vi "RT Inhibit Bus B - Single RT.vi"(8 "error in (no error)":errorcluster, 11 "1553 Unit Test in":refnum<class "Remote Terminal.lvclass">) -> (0 "error out":errorcluster, 3 "1553 Unit Test out":refnum<class "Remote Terminal.lvclass">)   [LabVIEW 2020, in "Unit Tests.lvlib" / "Remote Terminal.lvclass"]
uses:
  Remote Terminal.lvclass
  Remote Terminal/TypeDefs/RT Configuration.ctl
  Remote Terminal/TypeDefs/RT-RT Timeout.ctl
  Remote Terminal/TypeDefs/Mode Code 17 Sync Configuration.ctl
  Remote Terminal/TypeDefs/RT Timetag Configuration.ctl
  Remote Terminal/TypeDefs/RT Command Config.ctl
  Frames & Messages/TypeDefs/Command Type.ctl
  Frames & Messages/TypeDefs/Command SubAddress.ctl
  Frames & Messages/TypeDefs/Command Word Count.ctl
  Frames & Messages/TypeDefs/Simplified Parameter Data Table.ctl
  Frames & Messages/TypeDefs/Scaling Information.ctl
  Remote Terminal.lvclass/Remote Terminal.ctl
  Remote Terminal/Remote Terminal.lvclass
  C:/Users/MattJ/Desktop/git/bci-1553-labview-api/src/1553 SubComponent/1553 SubComponent.lvclass
  <vilib>/addons/_JKI Toolkits/Caraya/classes/Assert/Assert True.vi
  1553 Session/1553 Session.lvclass
  Dependencies/FPGA Interface/FPGA Interface.lvclass
  <vilib>/addons/_JKI Toolkits/Caraya/classes/Test/Test.lvclass
  BCI-1553 API.lvlib
  1553 Component/1553 Component.lvclass
  <vilib>/addons/_JKI Toolkits/Caraya/classes/Assert/Assert.lvclass
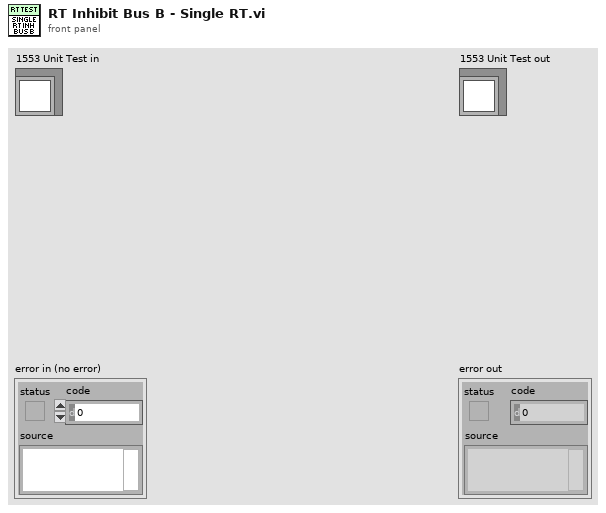
[diagram p1: front panel]
types:
  T1 = typedef "BCI-1553 API.lvlib/Remote Terminal.lvclass/RT Command Config.ctl" = cluster{"Command Type":T2, "SubAddress":T3, "Word Count\\Mode Code":T4, "Initial Data":u16[], "Data Fields":T5[]}
  T2 = typedef "BCI-1553 API.lvlib/Command Type.ctl" = enum16{"Transmit", "Receive"}
  T3 = typedef "BCI-1553 API.lvlib/Command SubAddress.ctl" = enum16{"Mode Code", "1", "2", "3", "4", "5", "6", "7", "8", "9", "10", "11", "12", "13", "14", "15", "16", "17", "18", "19", "20", "21", "22", "23", "24", "25", "26", "27", "28", "29", "30"}
  T4 = typedef "BCI-1553 API.lvlib/Command Word Count.ctl" = enum16{"1", "2", "3", "4", "5", "6", "7", "8", "9", "10", "11", "12", "13", "14", "15", "16", "17", "18", "19", "20", "21", "22", "23", "24", "25", "26", "27", "28", "29", "30", "31", "32"}
  T5 = typedef "BCI-1553 API.lvlib/Simplified Parameter Data Table.ctl" = cluster{"Parameter Name":string, "Base Word":u16, "Scaling Info":T6}
  T6 = typedef "BCI-1553 API.lvlib/Scaling Information.ctl" = cluster{"Bit Offset":i32, "Bit Count":i32, "LSB Resolution":dbl, "2's Complement":bool, "Big Endian":bool, "Sign Bit":bool}
  T7 = typedef "BCI-1553 API.lvlib/Remote Terminal.lvclass/RT Configuration.ctl" = cluster{"RT-RT Timeout":T8, "Inhibit Bus A":bool, "Inhibit Bus B":bool, "Broadcast CMD Invalid":bool, "UnDef MCs Invalid":bool, "Notice 2 Data Storage":bool, "SMCP":bool, "Temp RX Buffer":bool, "Alt BIT Enable":bool, "Auto Bus Shutdown":bool, "MC 16 SR Reset":bool, "MC 17 Sync":T9, "MC 8 Reset":bool, "Remote Terminal Timetag Config":T10}
  T8 = typedef "BCI-1553 API.lvlib/Remote Terminal.lvclass/RT-RT Timeout.ctl" = enum16{"57us", "62us", "100us", "180us"}
  T9 = typedef "BCI-1553 API.lvlib/Remote Terminal.lvclass/Mode Code 17 Sync Configuration.ctl" = enum16{"Sync if Bit 0 = 1", "Sync if Bit 0 = 0", "Sync Unconditionally"}
  T10 = typedef "BCI-1553 API.lvlib/Remote Terminal.lvclass/RT Timetag Configuration.ctl" = enum16{"Disabled", "2us", "4us", "8us", "16us", "32us", "64us"}
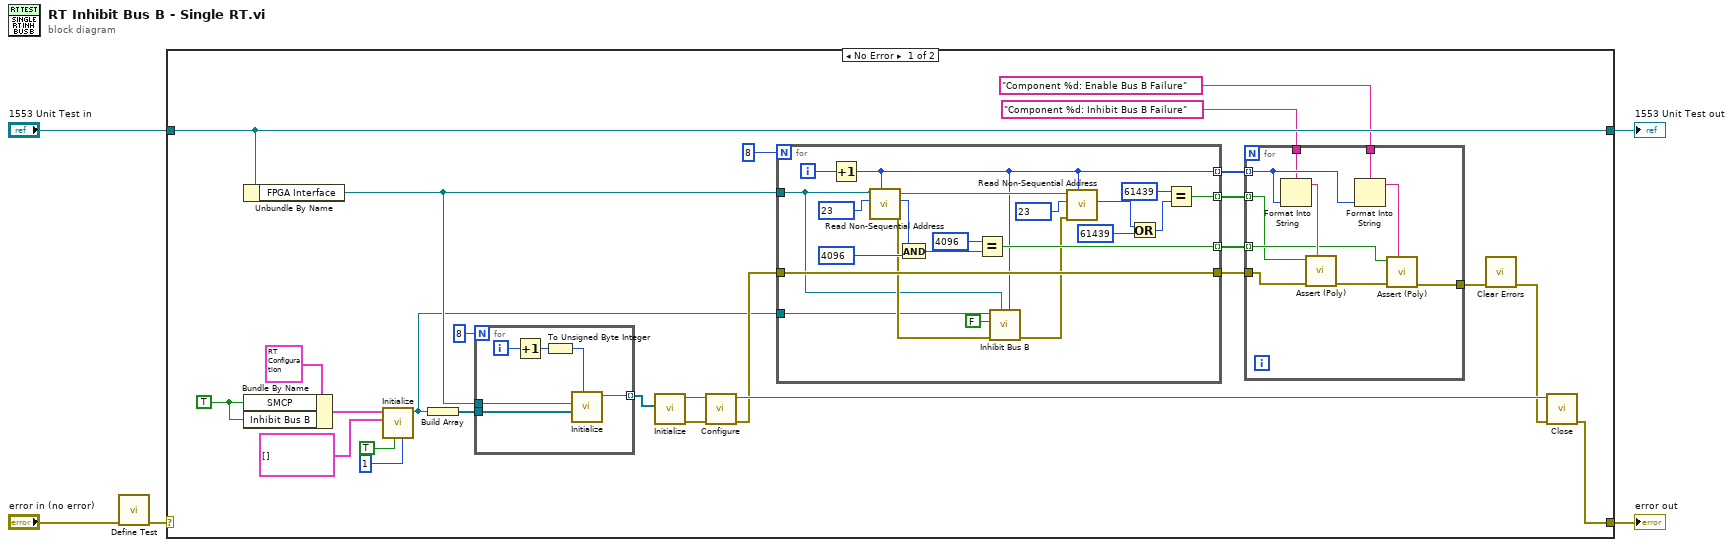
[diagram p0: block diagram]
diagram:
  n1 = call <vilib>:"Define Test.vi"("error in (no error)"="error in (no error)") -> ("error out"=w1:errorcluster)  [unwired: 9 in, 1 out]
  n2 = case shown="No Error" w1 {
    selector: w1 -> [_ w69]
    tunnel: [w14 w69] -> w5
    tunnel: [w25 w68] -> w3
    tunnel: "1553 Unit Test in" -> [w25 w68]
    frame No Error {
      w27 = TRUE ("SMCP")
      n3 = Unbundle By Name(w25) -> ("FPGA Interface"=w12:refnum<class "FPGA Interface.lvclass">)
      n4 = Bundle By Name(cluster=T7 {"RT-RT Timeout"=enum."57us", "Inhibit Bus A"=FALSE, "Inhibit Bus B"=FALSE, "Broadcast CMD Invalid"=FALSE, "UnDef MCs Invalid"=FALSE, "Notice 2 Data Storage"=FALSE, "SMCP"=FALSE, "Temp RX Buffer"=FALSE, "Alt BIT Enable"=FALSE, "Auto Bus Shutdown"=FALSE, "MC 16 SR Reset"=FALSE, "MC 17 Sync"=enum."Sync if Bit 0 = 1", "MC 8 Reset"=FALSE, "Remote Terminal Timetag Config"=enum."Disabled"} ("RT Configuration"), "SMCP"=w27, "Inhibit Bus B"=w27) -> (w30:T7)
      n5 = call "Initialize.vi"("Terminal Address"=u8 1 ("RT Address (0-30)"), "RT 1?"=TRUE, "RT Commands"=T1[] [], "RT Configuration"=w30) -> ("Remote Terminal out"=w10:refnum<class "Remote Terminal.lvclass">)  [unwired: 6 in, 1 out]
      n6 = Build Array(w10) -> (w23:refnum<class "Remote Terminal.lvclass">[])
      n7 = for {
        N: 8 -> [_]
        tunnel: [w65] -> w22 mode=indexing
        tunnel: w23 -> [w64]
        tunnel: w12 -> [w63]
        i -> [w67]
        n8 = Increment(x=w67) -> (x+1=w62:i32)
        n9 = To Unsigned Byte Integer(number=w62) -> (unsigned 8bit integer=w66:u8)
        n10 = call "Initialize.vi"("Component ID (1-8)"=w66, "SubComponents"=w64, "FPGA Interface"=w63) -> ("1553 Component out"=w65:refnum<class "1553 Component.lvclass">)  [unwired: 7 in, 1 out]
      }
      n11 = call "Initialize.vi"("Components"=w22) -> ("error out"=w20:errorcluster, "1553 Board out"=w21:refnum<class "1553 Session.lvclass">)  [unwired: 9 in]
      n12 = call-dynamic "Configure.vi"("error in (no error)"=w20, "1553 Board in"=w21) -> ("error out"=w11:errorcluster, "1553 Board out"=w17:refnum<class "1553 Session.lvclass">)  [unwired: 8 in]
      n13 = for {
        N: 8 -> [_]
        tunnel: w11 -> [w45]
        tunnel: [w45] -> w9
        tunnel: w12 -> [w40]
        tunnel: [w44] -> w8 mode=indexing
        tunnel: [w39] -> w6 mode=indexing
        tunnel: w10 -> [w42]
        tunnel: [w35] -> w7 mode=indexing
        i -> [w46]
        n14 = Increment(x=w46) -> (x+1=w39:i32)
        n15 = call-dynamic "Read Non-Sequential Address.vi"("Target IC (1-8)"=w39, "Address"=u16 23, "FPGA Interface in"=w40) -> ("error out"=w43:errorcluster, "Data"=w47:u16)  [unwired: 7 in]
        n16 = And(x=w47, y=u16 4096) -> (x .and. y?=w48:u16)
        n17 = Equal?(x=u16 4096, y=w48) -> (x = y?=w44:bool)
        n18 = call-dynamic "Inhibit Bus B.vi"("Component ID"=w39, "FPGA Interface"=w40, "error in (no error)"=w43, "Bus B Inhibited?"=FALSE ("Inhibit Bus A?"), "Remote Terminal in"=w42) -> ("error out"=w36:errorcluster)  [unwired: 5 in, 1 out]
        n19 = call-dynamic "Read Non-Sequential Address.vi"("Target IC (1-8)"=w39, "error in (no error)"=w36, "Address"=u16 23, "FPGA Interface in"=w40) -> ("Data"=w33:u16)  [unwired: 6 in, 1 out]
        n20 = Or(x=w33, y=u16 61439) -> (x .or. y?=w32:u16)
        n21 = Equal?(x=u16 61439, y=w32) -> (x = y?=w35:bool)
      }
      n22 = for {
        tunnel: w6 -> [w59] mode=indexing
        tunnel: w8 -> [w58] mode=indexing
        tunnel: w7 -> [w57] mode=indexing
        tunnel: "Component %d: Inhibit Bus B Failure" ("custom report message (\"\")") -> [w56]
        tunnel: "Component %d: Enable Bus B Failure" ("custom report message (\"\")") -> [w55]
        tunnel: w9 -> [w54]
        tunnel: [w52] -> w15
        n23 = Format Into String(format string=w56, w59) -> (resulting string=w61:string)  [unwired: 2 in, 1 out]
        n24 = call-poly <vilib>:"Assert (Poly).vi"("Label"=w61, "error in (no error)"=w54, "True?"=w57) -> ("error out"=w53:errorcluster)  [unwired: 7 in, 1 out]
        n25 = Format Into String(format string=w55, w59) -> (resulting string=w60:string)  [unwired: 2 in, 1 out]
        n26 = call-poly <vilib>:"Assert (Poly).vi"("Label"=w60, "error in (no error)"=w53, "True?"=w58) -> ("error out"=w52:errorcluster)  [unwired: 7 in, 1 out]
      }
      n27 = call <vilib>:"Clear Errors.vi"("error in (no error)"=w15) -> ("error out"=w16:errorcluster)  [unwired: 5 in, 1 out]
      n28 = call-dynamic "Close.vi"("error in (no error)"=w16, "1553 Board in"=w17) -> ("error out"=w14:errorcluster)  [unwired: 9 in]
    }
    frame Error {
    }
  }
  "error out" <- w5
  "1553 Unit Test out" <- w3
